vi "ROI entry-Get image size.vi"(8 "error in (no error)":errorcluster) -> (0 "error out":errorcluster, 3 "Image size":cluster{"X Resolution":i32, "Y Resolution":i32})   [LabVIEW 2017]
uses:
  <vilib>/vision/Image Controls.llb/IMAQ Image.ctl
  Globals/gl_ROI Entry UI globals.vi
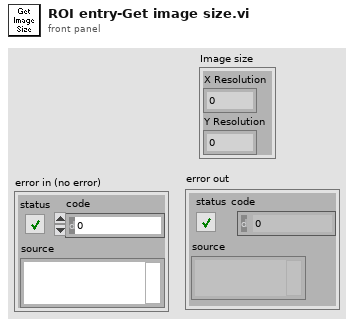
[diagram p1: front panel]
types:
  T1 = typedef "IMAQ Image.ctl" = refnum<image>
  T2 = typedef "ROI entry screen ctrl refs cluster.ctl" = cluster{"Done button":refnum<vi>, "Imaging button":refnum<vi>, "Acquisition button":refnum<vi>, "POI dwell time (us)":refnum<vi>, "Scan dwell time per pixel (us)":refnum<vi>, "# of planes":refnum<vi>, "Zoom Ctrl":refnum<vi>, "Equal size":refnum<vi>, "Channel":refnum<vi>, "Image Display":refnum<vi>, "Z-Plane Selector":refnum<vi>, "Number of lines left":refnum<vi>, "Z-stack folder path":refnum<vi>, "POI Density":refnum<vi>, "Arb Plane Entry":refnum<vi>, "Whole plane":refnum<vi>, "Clear Last":refnum<vi>, "Clear All":refnum<vi>, "Trial Length (sec)":refnum<vi>, "Palette Type":refnum<vi>, "Intensity slider":refnum<vi>, "# POI":refnum<vi>, "Max Z Proj":refnum<vi>, "Zplane ind":refnum<vi>, "Wavelength (nm)":refnum<vi>, "Number of Trials":refnum<vi>, "Funct stim.trig.enable":refnum<vi>, "Funct stim.trig.delay (s)":refnum<vi>, "Line Mode":refnum<vi>, "Step size (µm)":refnum<vi>, "ROI move mode":refnum<vi>, "Cool-down time (s)":refnum<vi>, "Enable cool-down time":refnum<vi>, "Motor Z ind. (um)":refnum<vi>, "AOL Z ind. (um)":refnum<vi>, "Load Reference Image":refnum<vi>}
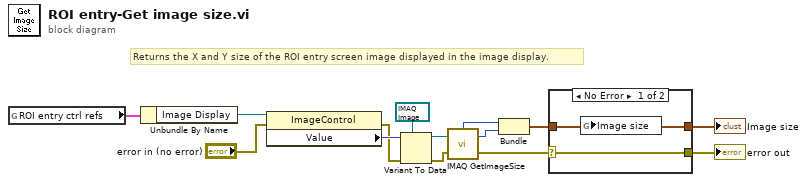
[diagram p0: block diagram]
diagram:
  # "Returns the X and Y size of the ROI entry screen image displayed in the image display."
  n1 = global read "gl_ROI Entry UI globals.vi" "ROI entry ctrl refs"() -> (w11:T2)
  n2 = Unbundle By Name(w11) -> ("Image Display"=w10:refnum<vi>)
  n3 = property on="Property Node" class="ImageControl"(reference=w10, error in="error in (no error)") -> (error out=w4:errorcluster, "Value"=w9:variant)  [unwired: 1 out]
  n4 = Variant To Data(error in=w4, type=T1 refnum ("element"), Variant=w9) -> (data=w7:T1, error out=w14:errorcluster)
  n5 = call "IMAQ GetImageSize"("Image"=w7, "error in (no error)"=w14) -> ("Y Resolution"=w13:i32, "X Resolution"=w12:i32, "error out"=w3:errorcluster)  [unwired: 2 in]
  n6 = Bundle("X Resolution"=w12, "Y Resolution"=w13) -> (w6:cluster{"X Resolution":i32, "Y Resolution":i32})  [unwired: 1 in]
  n7 = case shown="No Error" w3 {
    selector: w3 -> [w16 w18]
    tunnel: w6 -> [w15 w17]
    tunnel: [w16 w18] -> w2
    tunnel: [w15 w17] -> w1
    frame No Error {
      n8 = global write "gl_ROI Entry UI globals.vi" "Image size"(w15) -> ()
    }
    frame Error {
    }
  }
  "Image size" <- w1
  "error out" <- w2
